vi "indexed_cache_long.vi"(3 "bool":bool, 4 "start index":u8, 5 "index":u8) -> (1 "long":u64)   [LabVIEW 2018]
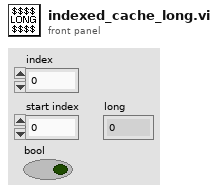
[diagram p1: front panel]
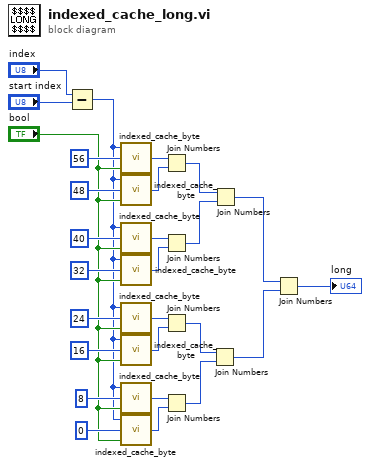
[diagram p0: block diagram]
diagram:
  n1 = Subtract(x="index", y="start index") -> (x-y=w2:u8)
  n2 = call "indexed_cache_byte.vi"("bool"="bool", "start_index"=u8 56, "index"=w2) -> ("bool_byte"=w18:u8)  [unwired: 2 in]
  n3 = call "indexed_cache_byte.vi"("bool"="bool", "start_index"=u8 48, "index"=w2) -> ("bool_byte"=w17:u8)  [unwired: 2 in]
  n4 = call "indexed_cache_byte.vi"("bool"="bool", "start_index"=u8 40, "index"=w2) -> ("bool_byte"=w15:u8)  [unwired: 2 in]
  n5 = call "indexed_cache_byte.vi"("bool"="bool", "start_index"=u8 32, "index"=w2) -> ("bool_byte"=w16:u8)  [unwired: 2 in]
  n6 = call "indexed_cache_byte.vi"("bool"="bool", "start_index"=u8 24, "index"=w2) -> ("bool_byte"=w14:u8)  [unwired: 2 in]
  n7 = call "indexed_cache_byte.vi"("bool"="bool", "start_index"=u8 16, "index"=w2) -> ("bool_byte"=w13:u8)  [unwired: 2 in]
  n8 = call "indexed_cache_byte.vi"("bool"="bool", "start_index"=u8 8, "index"=w2) -> ("bool_byte"=w12:u8)  [unwired: 2 in]
  n9 = call "indexed_cache_byte.vi"("bool"="bool", "start_index"=u8 0, "index"=w2) -> ("bool_byte"=w11:u8)  [unwired: 2 in]
  n10 = Join Numbers(hi=w18, lo=w17) -> ((hi.lo)=w10:u16)
  n11 = Join Numbers(hi=w15, lo=w16) -> ((hi.lo)=w9:u16)
  n12 = Join Numbers(hi=w14, lo=w13) -> ((hi.lo)=w8:u16)
  n13 = Join Numbers(hi=w12, lo=w11) -> ((hi.lo)=w7:u16)
  n14 = Join Numbers(hi=w8, lo=w7) -> ((hi.lo)=w5:u32)
  n15 = Join Numbers(hi=w10, lo=w9) -> ((hi.lo)=w6:u32)
  n16 = Join Numbers(hi=w6, lo=w5) -> ((hi.lo)=→"long":u64)
